vi "Initialize Daemon.vi"(8 "error in (no error)":errorcluster, 9 "data model":refnum<class "Device Data Model.lvclass">, 10 "transmission data unit":refnum<class "Transmission Data Unit.lvclass">, 11 "TCP slave in":refnum<class "TCP Slave.lvclass">) -> (0 "error out":errorcluster, 3 "TCP slave out":refnum<class "TCP Slave.lvclass">)   [LabVIEW 2020, in "SubVIs.lvlib" / "TCP Slave.lvclass"]
doc: "Launches the connection daemon and creates the notifier which will allow it to quit."
uses:
  <vilib>/Modbus/subvis/Protocol/TCP/TCP Slave/TCP Slave.lvclass
  <vilib>/Modbus/subvis/Transmission Data Unit (ADU)/Transmission Data Unit/Transmission Data Unit.lvclass
  <vilib>/Modbus/subvis/Data and Functions/Device Data Model/Device Data Model.lvclass
  <vilib>/Modbus/subvis/Protocol/TCP/TCP Slave/TCP Slave.lvclass/TCP Slave.ctl
  <vilib>/Modbus/subvis/Protocol/Interfaces/Network Slave/Network Slave.lvclass
  <vilib>/Modbus/subvis/SubVIs.lvlib
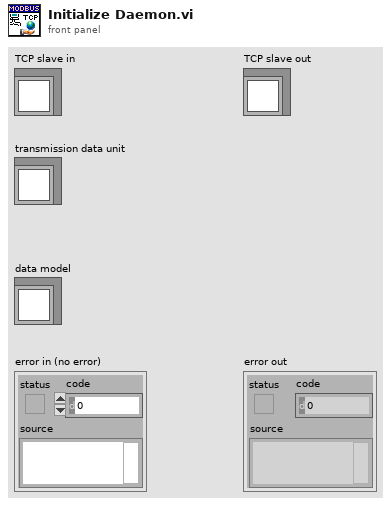
[diagram p1: front panel]
types:
  T1 = cluster{"Currently Connected":u32, "Connection Records":refnum<data-value>[]}
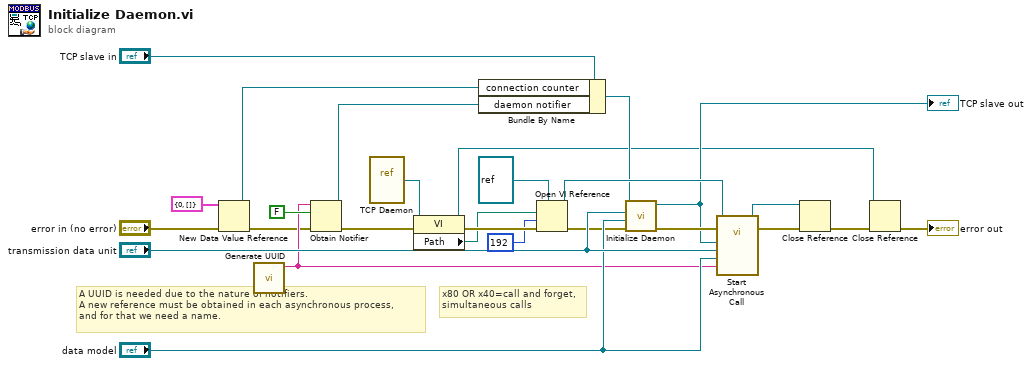
[diagram p0: block diagram]
diagram:
  # "x80 OR x40=call and forget,\nsimultaneous calls"
  # "A UUID is needed due to the nature of notifiers.\nA new reference must be obtained in each asynchronous process,\nand for that we need a name."
  n1 = New Data Value Reference(data value=T1 {"Currently Connected"=0, "Connection Records"=[]} ("Connection Counter"), error in="error in (no error)") -> (data value reference=w6:refnum<data-value>, error out=w7:errorcluster)
  n2 = call <vilib>:"Generate UUID.vi"() -> ("UUID"=w13:string)  [unwired: 11 in]
  n3 = Obtain Notifier(name (unnamed)=w13, notification data type=FALSE, error in (no error)=w7) -> (notifier out=w14:refnum<notifier>, error out=w16:errorcluster)  [unwired: 1 in, 1 out]
  n4 = vi-ref <vilib>:"TCP Daemon.vi"() -> (w22:refnum<vi>)
  n5 = property class="VI"(reference=w22, error in=w16) -> (reference out=w1:refnum<vi>, error out=w21:errorcluster, "Path"=w20:path)
  n6 = Bundle By Name(cluster="TCP slave in", "connection counter"=w6, "daemon notifier"=w14) -> (w11:refnum<class "TCP Slave.lvclass">)
  n7 = Open VI Reference(type specifier VI Refnum (for type only)=refnum<vi> refnum, vi path=w20, options=192 ("x .or. y?"), error in (no error)=w21) -> (vi reference=w19:refnum<vi>, error out=w10:errorcluster)  [unwired: 2 in]
  n8 = call-parent "Initialize Daemon.vi"("error in (no error)"=w10, "data model"="data model", "transmission data unit"="transmission data unit", "network slave in"=w11) -> ("error out"=w12:errorcluster, "network slave out"=w9:refnum<class "TCP Slave.lvclass">)  [unwired: 6 in]
  "TCP slave out" <- w9
  n9 = call-by-ref "Start Asynchronous Call"(reference=w19, error in=w12, "UUID"=w13, "Data Model"="data model", "transmission data unit"="transmission data unit", "TCP slave in"=w9) -> (reference out=w2:refnum<vi>, error out=w25:errorcluster)  [unwired: 8 in]
  n10 = Close Reference(reference=w2, error in (no error)=w25) -> (error out=w4:errorcluster)
  n11 = Close Reference(reference=w1, error in (no error)=w4) -> (error out=→"error out":errorcluster)
